vi "Practica 7 Alejandro Tejada ITIW31.vi"() -> ()   [LabVIEW 2018]
panel:
  out "Tamano de antena Marconi":dbl
  out "Tamano de antena Hertz":dbl
  in  "Frecuencia":dbl
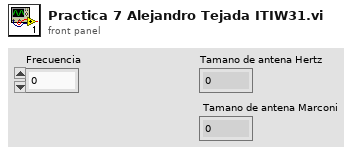
[diagram p1: front panel]
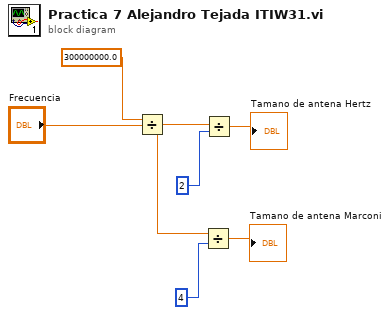
[diagram p0: block diagram]
diagram:
  n1 = Divide(x=300000000.0, y="Frecuencia") -> (x/y=w1:dbl)
  n2 = Divide(x=w1, y=4) -> (x/y=→"Tamano de antena Marconi":dbl)
  n3 = Divide(x=w1, y=2) -> (x/y=→"Tamano de antena Hertz":dbl)
